vi "Set Transfer Channels.vi"(8 "error in (no error)":errorcluster, 10 "channels":T1[](array[typedef]) {"string offset" format="%d bytes"}, 11 "transfer in":T4={"name"="Transfer", "byte order"=enum."big-endian", "settings"=[], "channels"=[]} {"channels"."string offset" format="%d bytes"}) -> (0 "error out":errorcluster, 3 "transfer out":T4={"name"="Transfer", "byte order"=enum."big-endian", "settings"=[], "channels"=[]} {"channels"."string offset" format="%d bytes"})   [LabVIEW 2017, in "DSF Core.lvlib" / "Configuration Session.lvclass"]
uses:
  Configuration Session.lvclass
  Typedefs/DSF Engine Transfer Configuration.ctl
  Typedefs/DSF Byte Order.ctl
  Typedefs/DSF Settings Info.ctl
  Typedefs/DSF Engine Channel Configuration.ctl
  Typedefs/DSF Data Type.ctl
  DSF Core.lvlib
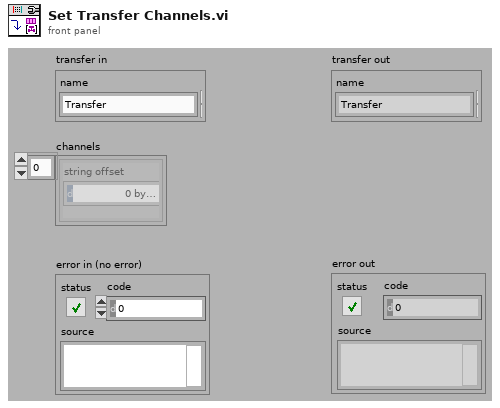
[diagram p1: front panel]
types:
  T1 = typedef "DSF Core.lvlib/DSF Engine Channel Configuration.ctl" = cluster{"string offset":u64, "string data type":T2, "engine data type":T2, "name":string, "settings":T3, "units":string}
  T2 = typedef "DSF Core.lvlib/DSF Data Type.ctl" = enum8{"Bool", "SGL", "DBL", "I8", "I16", "I32", "I64", "U8", "U16", "U32", "U64"}
  T3 = typedef "DSF Core.lvlib/DSF Settings Info.ctl" = cluster{"key":string, "value":string}[]
  T4 = typedef "DSF Core.lvlib/DSF Engine Transfer Configuration.ctl" = cluster{"name":string, "byte order":T5, "settings":T3, "channels":T1[]}
  T5 = typedef "DSF Core.lvlib/DSF Byte Order.ctl" = enum8{"big-endian", "little-endian"}
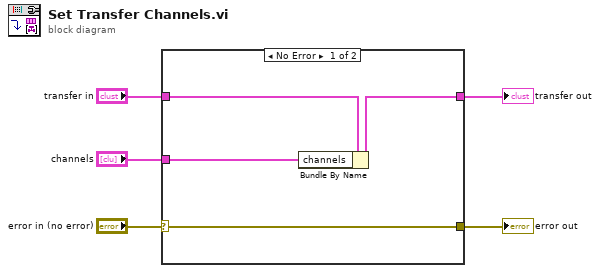
[diagram p0: block diagram]
diagram:
  n1 = case shown="No Error" "error in (no error)" {
    selector: "error in (no error)" -> [w7 w11]
    tunnel: [w7 w11] -> w5
    tunnel: [w8 w10] -> w3
    tunnel: "transfer in" -> [w9 w10]
    tunnel: "channels" -> [w6 _]
    frame No Error {
      n2 = Bundle By Name(cluster=w9, "channels"=w6) -> (w8:T4)
    }
    frame Error {
    }
  }
  "error out" <- w5
  "transfer out" <- w3
